vi "Planta_303_ver5.vi"() -> ()   [LabVIEW 2014]
uses:
  <vilib>/measure/NI_MABase.lvlib
panel:
  out "Waveform Chart 2":dynamicdata(graph)
  in  "Duty cycle (%)":dbl=50.0 format="%0.2f"
  out "Tanque":dbl(slide) scale=0.0..300.0
  in  "Escolha o Sinal":string(combo)
  out "Waveform Chart":waveform(dbl)(graph)
  in  "Amplitude":dbl=1.0
  in  "Frequency":dbl=10.1
  in  "Offset":dbl
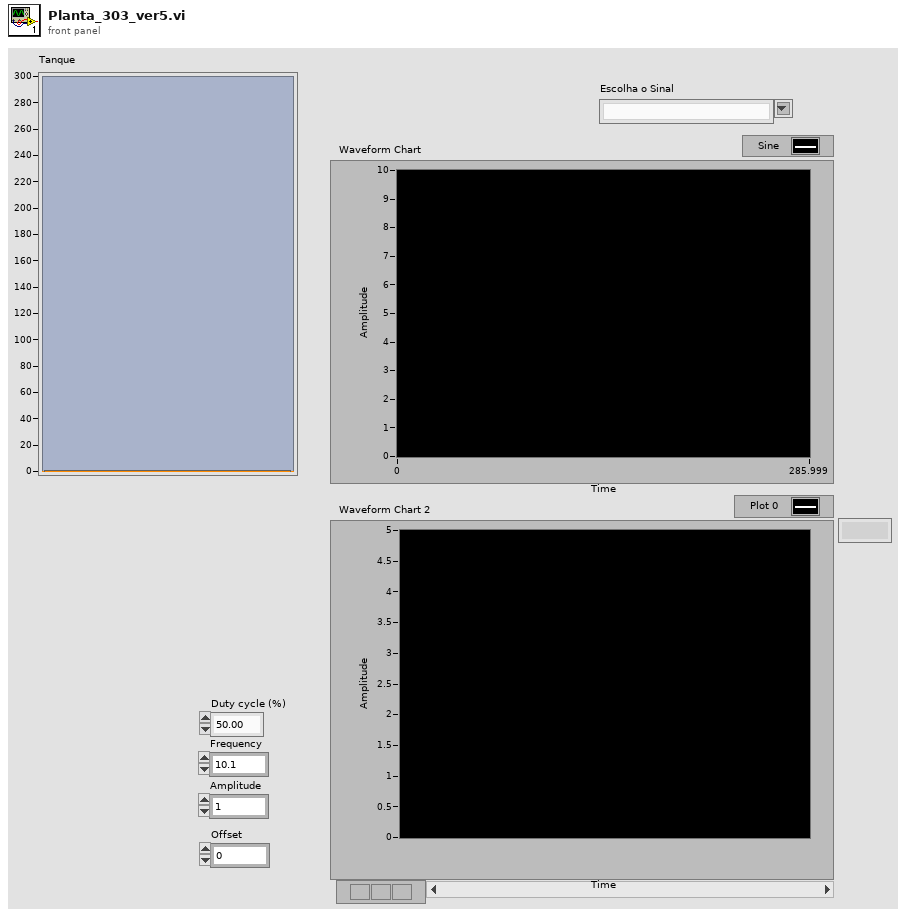
[diagram p1: front panel]
types:
  T1 = enum16{"Sine Wave", "Triangle Wave", "Square Wave", "Sawtooth Wave"}
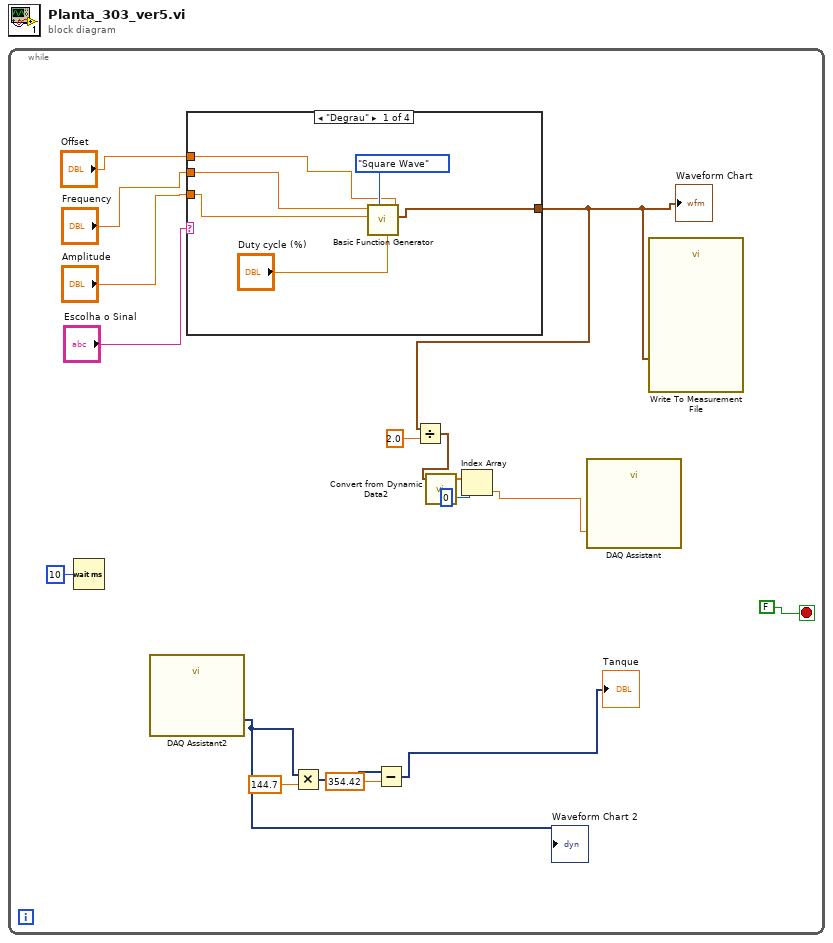
[diagram p0: block diagram]
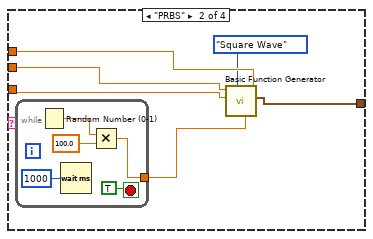
[diagram p2: hidden frame]
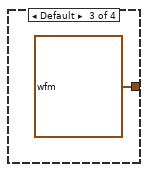
[diagram p3: hidden frame]
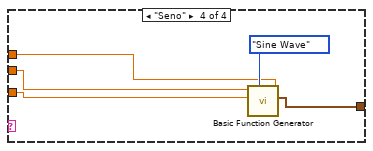
[diagram p4: hidden frame]
diagram:
  n1 = while {
    stop <- FALSE stop-if-true
    n2 = Wait (ms)(milliseconds to wait=u32 10) -> ()  [unwired: 1 out]
    n3 = call "DAQ Assistant2"() -> ("data"=w4:dynamicdata)  [unwired: 17 in, 2 out]
    "Waveform Chart 2" <- w4
    n4 = case shown="\"Degrau\"" "Escolha o Sinal" {
      tunnel: "Offset" -> [w22 w27 _ w39]
      tunnel: "Frequency" -> [w21 w26 _ w38]
      tunnel: "Amplitude" -> [w20 w28 _ w37]
      tunnel: [w19 w29 waveform(dbl) {"t0"=timestamp(0 s since 1904-01-01), "dt"=1.0, "Y"=[]} ("signal out") w36] -> w10
      frame "Degrau" {
        n5 = call <vilib>:"Basic Function Generator.vi"("offset"=w22, "square wave duty cycle (%)"="Duty cycle (%)", "signal type"=T1."Square Wave", "amplitude"=w20, "frequency"=w21) -> ("signal out"=w19:waveform(dbl))  [unwired: 4 in, 2 out]
      }
      frame "PRBS" {
        n6 = while {
          tunnel: [w33] -> w25
          stop <- TRUE stop-if-true
          n7 = Random Number (0-1)() -> (number: 0 to 1=w34:dbl)
          n8 = Wait (ms)(milliseconds to wait=u32 1000) -> ()  [unwired: 1 out]
          n9 = Multiply(x=w34, y=100.0) -> (x*y=w33:dbl)
        }
        n10 = call <vilib>:"Basic Function Generator.vi"("offset"=w27, "square wave duty cycle (%)"=w25, "signal type"=T1."Square Wave", "amplitude"=w28, "frequency"=w26) -> ("signal out"=w29:waveform(dbl))  [unwired: 4 in, 2 out]
      }
      frame Default {
      }
      frame "Seno" {
        n11 = call <vilib>:"Basic Function Generator.vi"("offset"=w39, "signal type"=T1."Sine Wave", "amplitude"=w37, "frequency"=w38) -> ("signal out"=w36:waveform(dbl))  [unwired: 5 in, 2 out]
      }
    }
    "Waveform Chart" <- w10
    n12 = Multiply(x=w4, y=144.7) -> (x*y=w3:dynamicdata)
    n13 = Subtract(x=w3, y=354.42) -> (x-y=→"Tanque":dynamicdata)
    n14 = Divide(x=w10, y=2.0) -> (x/y=w7:waveform(dbl))
    n15 = call "Convert from Dynamic Data2"("Dynamic Data Type"=w7) -> ("Array"=w9:dbl[])  [unwired: 3 in]
    n16 = Index Array "Index Array"(array=w9, index=0) -> (element=w6:dbl)
    n17 = call "DAQ Assistant"("data"=w6) -> ()  [unwired: 17 in, 2 out]
    n18 = call "Write To Measurement File"("Signals"=w10) -> ()  [unwired: 16 in, 3 out]
  }
